vi "Post-Build Action.vi"(5 "Files Generated by Build":path[](array[path]), 6 "Top Level/Always Included VIs":path[](array[path]), 7 "Destination Path":path, 8 "error in (no error)":errorcluster, 9 "Target Name":string, 10 "Build Specification Name":string, 11 "Project Path":path) -> (0 "error out":errorcluster)   [LabVIEW 2025, in "Automotive Vision UI.lvlib"]
uses:
  Automotive Vision UI.lvlib
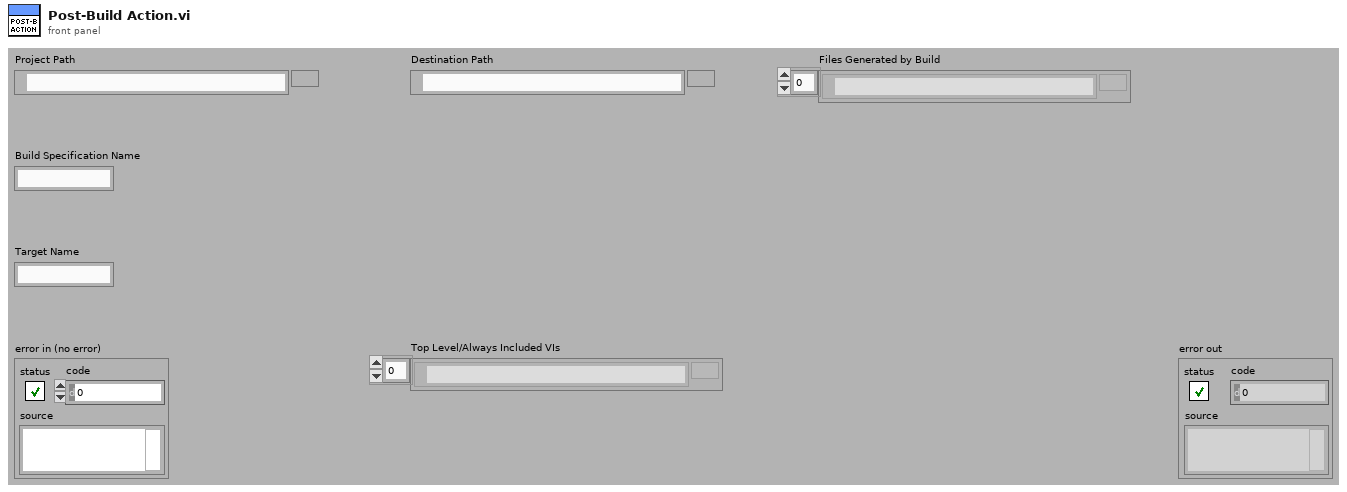
[diagram p1: front panel]
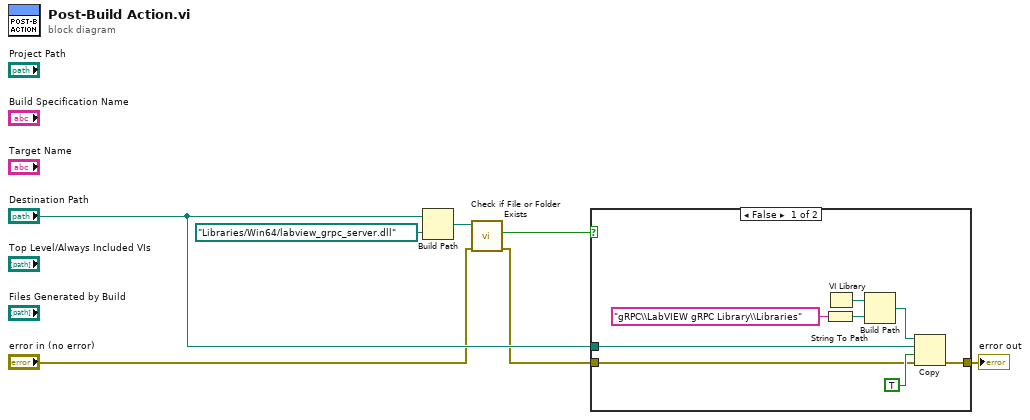
[diagram p0: block diagram]
diagram:
  n1 = Build Path(base path="Destination Path", name or relative path=path "Libraries/Win64/labview_grpc_server.dll") -> (appended path=w5:path)
  n2 = call <vilib>:"Check if File or Folder Exists.vi"("error in (no error)"="error in (no error)", "path"=w5) -> ("error out"=w1:errorcluster, "file or folder exists?"=w3:bool)  [unwired: 7 in, 1 out]
  n3 = case shown="False" w3 {
    tunnel: [w11 w16] -> w7
    tunnel: w1 -> [w10 w16]
    tunnel: "Destination Path" -> [w8 _]
    frame False {
      n4 = String To Path(string="gRPC\\LabVIEW gRPC Library\\Libraries") -> (path=w14:path)
      n5 = VI Library() -> (path=w15:path)
      n6 = Build Path(base path=w15, name or relative path=w14) -> (appended path=w13:path)
      n7 = Copy(8:w10, 9:TRUE ("overwrite (F)"), 10:w8, 11:w13) -> (0:w11:errorcluster)  [unwired: 1 in, 2 out]
    }
    frame True {
    }
  }
  "error out" <- w7
